vi "NTC Thermistor lookup.vi"(1 "Voltage Out":dbl) -> (0 "Temperature °C":dbl)   [LabVIEW 2024]
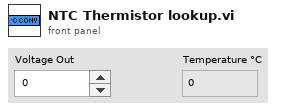
[diagram p1: front panel]
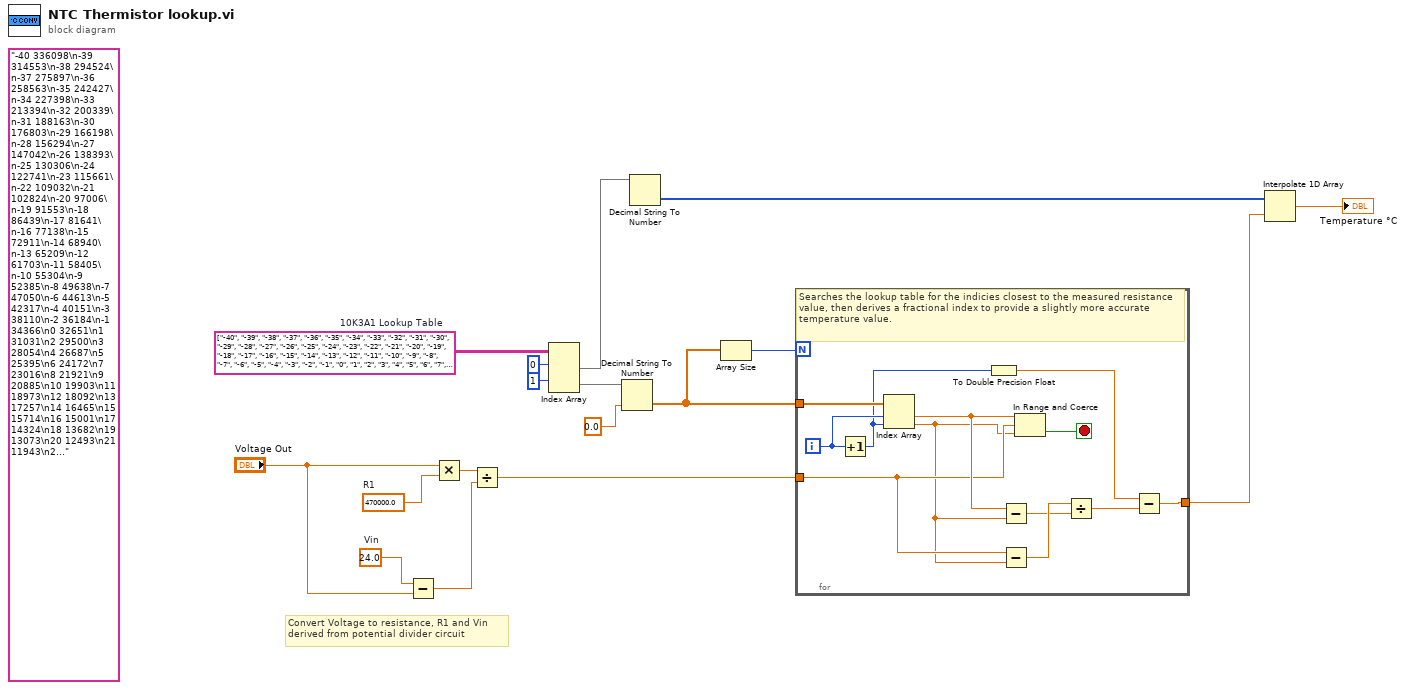
[diagram p0: block diagram]
diagram:
  w4 = 24.0  # Vin
  w3 = 470000.0  # R1
  w10 = string[][] [["-40", "-39", "-38", "-37", "-36", "-35", "-34", "-33", "-32", "-31", "-30", "-29", "-28", "-27", "-26", "-25", "-24", "-23", "-22", "-21", "-20", "-19", "-18", "-17", "-16", "-15", "-14", "-13", "-12", "-11", "-10", "-9", "-8", "-7", "-6", "-5", "-4", "-3", "-2", "-1", "0", "1", "2", "3", "4", "5", "6", "7", "8", "9", "10", "11", "12", "13", "14", "15", "16", "17", "18", "19", "20", "21", "22", "23", "24", "25", "26", "27", "28", "29", "30", "31", "32", "33", "34", "35", "36", "37", "38", "39", "40", "41", "42", "43", "44", "45", "46", "47", "48", "49", "50", "51", "52", "53", "54", "55", "56", "57", "58", "59", "60", "61", "62", "63", "64", "65", "66", "67", "68", "69", "70", "71", "72", "73", "74", "75", "76", "77", "78", "79", "80", "81", "82", "83", "84", "85", "86", "87", "88", "89", "90", "91", "92", "93", "94", "95", "96", "97", "98", "99", "100", "101", "102", "103", "104", "105", "106", "107", "108", "109", "110", "111", "112", "113", "114", "115", "116", "117", "118", "119", "120", "121", "122", "123", "124", "125"], ["336098", "314553", "294524", "275897", "258563", "242427", "227398", "213394", "200339", "188163", "176803", "166198", "156294", "147042", "138393", "130306", "122741", "115661", "109032", "102824", "97006", "91553", "86439", "81641", "77138", "72911", "68940", "65209", "61703", "58405", "55304", "52385", "49638", "47050", "44613", "42317", "40151", "38110", "36184", "34366", "32651", "31031", "29500", "28054", "26687", "25395", "24172", "23016", "21921", "20885", "19903", "18973", "18092", "17257", "16465", "15714", "15001", "14324", "13682", "13073", "12493", "11943", "11420", "10923", "10450", "10000", "9572", "9165", "8777", "8408", "8056", "7721", "7402", "7097", "6807", "6530", "6266", "6014", "5774", "5544", "5325", "5116", "4916", "4724", "4542", "4367", "4200", "4040", "3887", "3741", "3601", "3467", "3339", "3216", "3098", "2985", "2877", "2773", "2674", "2579", "2487", "2399", "2315", "2234", "2157", "2082", "2011", "1942", "1876", "1813", "1752", "1693", "1637", "1582", "1530", "1480", "1432", "1385", "1341", "1298", "1256", "1216", "1178", "1141", "1105", "1070", "1037", "1005", "974", "945", "916", "888", "862", "836", "811", "787", "764", "741", "720", "699", "678", "659", "640", "622", "604", "587", "571", "555", "539", "524", "510", "496", "482", "469", "457", "444", "432", "421", "410", "399", "388", "378", "368", "359", "350", "341"]]  # 10K3A1 Lookup Table
  (unwired) "-40 336098\n-39 314553\n-38 294524\n-37 275897\n-36 258563\n-35 242427\n-34 227398\n-33 213394\n-32 200339\n-31 188163\n-30 176803\n-29 166198\n-28 156294\n-27 147042\n-26 138393\n-25 130306\n-24 122741\n-23 115661\n-22 109032\n-21 102824\n-20 97006\n-19 91553\n-18 86439\n-17 81641\n-16 77138\n-15 72911\n-14 68940\n-13 65209\n-12 61703\n-11 58405\n-10 55304\n-9 52385\n-8 49638\n-7 47050\n-6 44613\n-5 42317\n-4 40151\n-3 38110\n-2 36184\n-1 34366\n0 32651\n1 31031\n2 29500\n3 28054\n4 26687\n5 25395\n6 24172\n7 23016\n8 21921\n9 20885\n10 19903\n11 18973\n12 18092\n13 17257\n14 16465\n15 15714\n16 15001\n17 14324\n18 13682\n19 13073\n20 12493\n21 11943\n22 11420\n23 10923\n24 10450\n25 10000\n26 9572\n27 9165\n28 8777\n29 8408\n30 8056\n31 7721\n32 7402\n33 7097\n34 6807\n35 6530\n36 6266\n37 6014\n38 5774\n39 5544\n40 5325\n41 5116\n42 4916\n43 4724\n44 4542\n45 4367\n46 4200\n47 4040\n48 3887\n49 3741\n50 3601\n51 3467\n52 3339\n53 3216\n54 3098\n55 2985\n56 2877\n57 2773\n58 2674\n59 2579\n60 2487\n61 2399\n62 2315\n63 2234\n64 2157\n65 2082\n66 2011\n67 1942\n68 1876\n69 1813\n70 1752\n71 1693\n72 1637\n73 1582\n74 1530\n75 1480\n76 1432\n77 1385\n78 1341\n79 1298\n80 1256\n81 1216\n82 1178\n83 1141\n84 1105\n85 1070\n86 1037\n87 1005\n88 974\n89 945\n90 916\n91 888\n92 862\n93 836\n94 811\n95 787\n96 764\n97 741\n98 720\n99 699\n100 678\n101 659\n102 640\n103 622\n104 604\n105 587\n106 571\n107 555\n108 539\n109 524\n110 510\n111 496\n112 482\n113 469\n114 457\n115 444\n116 432\n117 421\n118 410\n119 399\n120 388\n121 378\n122 368\n123 359\n124 350\n125 341\n"
  # "Convert Voltage to resistance, R1 and Vin \nderived from potential divider circuit"
  n1 = Subtract(x=w4, y="Voltage Out") -> (x-y=w6:dbl)
  n2 = Multiply(x="Voltage Out", y=w3) -> (x*y=w5:dbl)
  n3 = Divide(x=w5, y=w6) -> (x/y=w1:dbl)
  n4 = Index Array(array=w10, index (row) #1=0 ("index (row)"), index (row) #2=1 ("index (row)")) -> (element #1=w9:string[], element #2=w8:string[])  [unwired: 2 in]
  n5 = Decimal String To Number(string=w8, default (0L)=0.0) -> (number=w15:dbl[])  [unwired: 1 in, 1 out]
  n6 = Decimal String To Number(string=w9) -> (number=w14:i32[])  [unwired: 2 in, 1 out]
  n7 = Array Size(array=w15) -> (size(s)=w16:i32)
  n8 = for {
    N: w16 -> [_]
    tunnel: w15 -> [w29]
    tunnel: w1 -> [w26]
    tunnel: [w20] -> w12
    i -> [w22]
    stop <- w28 stop-if-true
    # "Searches the lookup table for the indicies closest to the measured resistance value, then derives a fractional index to provide a slightly more accurate temperature value."
    n9 = Increment(x=w22) -> (x+1=w19:i32)
    n10 = Index Array(array=w29, index #1=w22, index #2=w19) -> (element #1=w27:dbl, element #2=w25:dbl)
    n11 = To Double Precision Float(number=w19) -> (double precision float=w18:dbl)
    n12 = Subtract(x=w27, y=w25) -> (x-y=w23:dbl)
    n13 = Subtract(x=w26, y=w25) -> (x-y=w24:dbl)
    n14 = In Range and Coerce(upper limit=w27, x=w26, lower limit=w25) -> (In Range?=w28:bool)  [unwired: 1 out]
    n15 = Divide(x=w24, y=w23) -> (x/y=w21:dbl)
    n16 = Subtract(x=w18, y=w21) -> (x-y=w20:dbl)
  }
  n17 = Interpolate 1D Array(1:w12, 2:w14) -> (0:→"Temperature °C":dbl)
